vi "Timekeeper.vi"   [LabVIEW 2011, in "EPS_Timekeeper.lvlib"]
uses:
  <vilib>/addons/Electrical Power/Example Support/PMU/Time Keeper/EPS_Timekeeper.lvlib
  <vilib>/addons/Electrical Power/Example Support/PMU/Time Keeper/timekeeper locked (g).vi
  <vilib>/addons/Electrical Power/Example Support/PMU/Time Keeper/timekeeper offset from timeref (g).vi
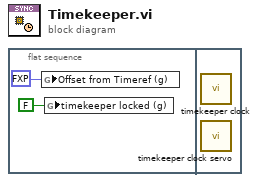
[diagram p0: block diagram]
diagram:
  n1 = flat-sequence {
    frame #0 {
      n2 = global write "timekeeper offset from timeref (g).vi" "Offset from Timeref (g)"(fxp<+/-,18,18> 0.0 ("Offset from Timeref (g)")) -> ()
      n3 = global write "timekeeper locked (g).vi" "timekeeper locked (g)"(FALSE ("timekeeper locked (g)")) -> ()
    }
    frame #1 {
      n4 = call <vilib>:"timekeeper clock.vi"() -> ()  [unwired: 12 in]
      n5 = call <vilib>:"timekeeper clock servo.vi"() -> ()  [unwired: 12 in]
    }
  }
